vi "Fetch Value.vi"(7 "PV name":string, 8 "error in":errorcluster, 11 "Source in":refnum<class "Source.lvclass">) -> (0 "error out":errorcluster, 2 "Value out":refnum<class "Value.lvclass">, 3 "Source out":refnum<class "Source.lvclass">)   [LabVIEW 2020, in "Server.lvlib" / "Source.lvclass"]
uses:
  Source.lvclass
  Value/Value/Value.lvclass
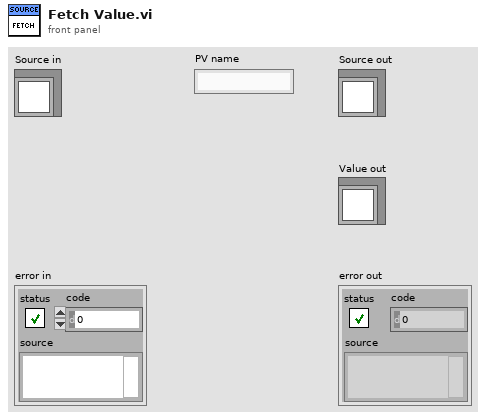
[diagram p1: front panel]
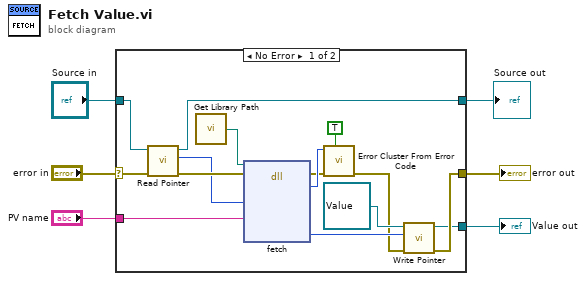
[diagram p0: block diagram]
diagram:
  n1 = case shown="No Error" "error in" {
    selector: "error in" -> [w21 w23]
    tunnel: [w9 w23] -> w5
    tunnel: [w17 w22] -> w1
    tunnel: "PV name" -> [w16 _]
    tunnel: [w8 _] -> w3
    tunnel: "Source in" -> [w7 w22]
    frame No Error {
      n2 = call-dynamic "Read Pointer.vi"("error in (no error)"=w21, "Source in"=w7) -> ("error out"=w20:errorcluster, "source pointer"=w18:i64, "Source out"=w17:refnum<class "Source.lvclass">)  [unwired: 7 in]
      n3 = call "Get Library Path.vi"() -> ("Path"=w19:path)  [unwired: 1 in]
      n4 = dll-call lib="?" fn="fetch"(path in=w19, error in=w20, "source"=w18, "pv_name"=w16) -> (error out=w13:errorcluster, "ret_code"=w14:i32, "value"=w11:i64)  [unwired: 4 in, 1 out]
      n5 = call <vilib>:"Error Cluster From Error Code.vi"("show call chain? (False)"=TRUE, "error in (no error)"=w13, "error code (0)"=w14) -> ("error out"=w10:errorcluster)  [unwired: 6 in]
      n6 = call-dynamic "Write Pointer.vi"("error in (no error)"=w10, "Pointer"=w11, "Value in"=refnum<class "Value.lvclass"> refnum) -> ("error out"=w9:errorcluster, "Value out"=w8:refnum<class "Value.lvclass">)  [unwired: 7 in]
    }
    frame Error {
    }
  }
  "error out" <- w5
  "Value out" <- w3
  "Source out" <- w1
